vi "Web Messaging.vi"   [LabVIEW 2013]
uses:
  <vilib>/Platform/browser.llb/Open URL in Default Browser (string).vi
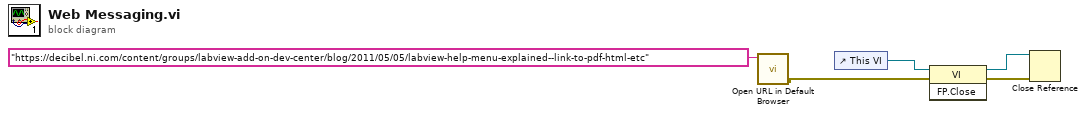
[diagram p0: block diagram]
diagram:
  n1 = call-poly <vilib>:"Open URL in Default Browser.vi"("URL"="https://decibel.ni.com/content/groups/labview-add-on-dev-center/blog/2011/05/05/labview-help-menu-explained--link-to-pdf-html-etc") -> ("error out"=w1:errorcluster)  [unwired: 5 in, 1 out]
  n2 = control-ref of="This VI"() -> (w2:refnum<vi>)
  n3 = invoke class="VI" method="FP.Close"(reference=w2, error in=w1) -> (reference out=w4:refnum<vi>, error out=w3:errorcluster)  [unwired: 1 in, 1 out]
  n4 = Close Reference(reference=w4, error in (no error)=w3) -> ()  [unwired: 1 out]
